vi "p1.vi"() -> ()   [LabVIEW 2023, in "d21.lvlib"]
uses:
  d21.lvlib
  AOC/AOC.lvlib
panel:
  out "Answer":i32
  in  "Example":string="...........\n.....###.#.\n.###.##..#.\n..#.#...#..\n....#.#....\n.##..S####.\n.##..#...#.\n.......##..\n.##.#.####.\n.##..##.##.\n..........."
  in  "Example":bool
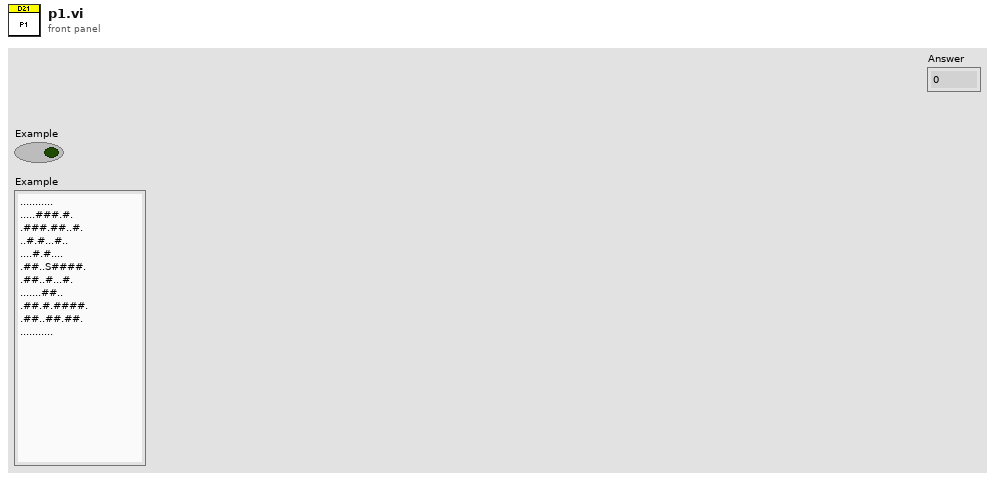
[diagram p1: front panel]
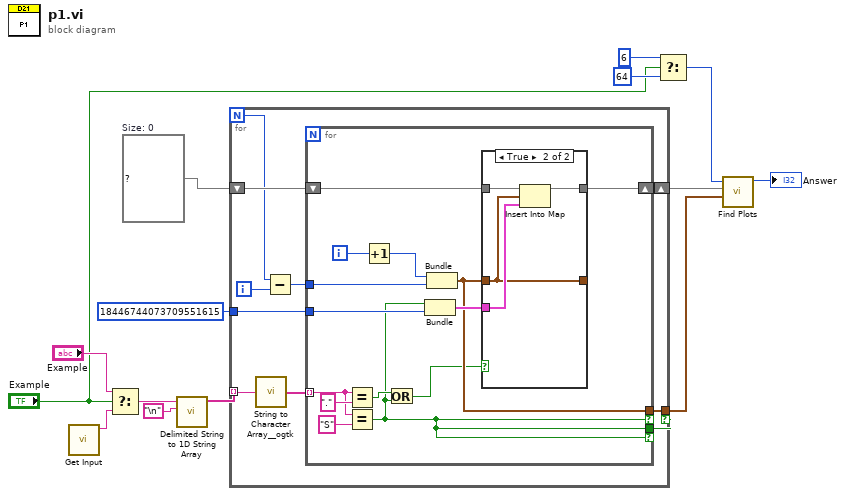
[diagram p0: block diagram]
diagram:
  w8 = map{cluster{i32, i32}, cluster{bool, u64}} {}  # Size: 0
  n1 = call "Get Input.vi"() -> ("Input"=w14:string)  [unwired: 11 in]
  n2 = Select(t="Example", s="Example", f=w14) -> (s? t:f=w13:string)
  n3 = call <vilib>:"Delimited String to 1D String Array.vi"("delimiter"="\n", "delimited string"=w13) -> ("string array"=w10:string[])  [unwired: 9 in]
  n4 = for {
    N -> [w15]
    tunnel: w10 -> [w24] mode=indexing
    tunnel: [w21] -> w3 if=w20
    tunnel: u64 18446744073709551615 -> [w19]
    shift-right: [w17] -> w4
    shift-left: w8 -> [w18]
    i -> [w22]
    n5 = call <userlib>:"String to Character Array__ogtk.vi"("Input String"=w24) -> ("Character Array"=w23:string[])
    n6 = Subtract(x=w15, y=w22) -> (x-y=w16:i32)
    n7 = for {
      tunnel: w23 -> [w37] mode=indexing
      tunnel: w16 -> [w34]
      tunnel: [w28] -> w21 if=w26
      tunnel: [w26] -> w20 if=w26
      tunnel: w19 -> [w33]
      shift-right: [w32] -> w17
      shift-left: w18 -> [w31]
      i -> [w35]
      n8 = Equal?(x=w37, y=".") -> (x = y?=w27:bool)
      n9 = Equal?(x=w37, y="S") -> (x = y?=w26:bool)
      n10 = Increment(x=w35) -> (x+1=w29:i32)
      n11 = Or(x=w27, y=w26) -> (x .or. y?=w25:bool)
      n12 = Bundle(w26, w33) -> (w30:cluster{bool, u64})  [unwired: 1 in]
      n13 = Bundle(w29, w34) -> (w28:cluster{i32, i32})  [unwired: 1 in]
      n14 = case shown="True" w25 {
        tunnel: [w40 w44] -> w32
        tunnel: w31 -> [w40 w43]
        tunnel: w28 -> [w39 w41]
        tunnel: w30 -> [_ w42]
        tunnel: [w39 w41] -> _
        frame False {
        }
        frame True {
          n15 = Insert Into Map(map in=w43, key=w41, value=w42) -> (map out=w44:map{cluster{i32, i32}, cluster{bool, u64}})  [unwired: 2 out]
        }
      }
    }
  }
  n16 = Select(t=6, s="Example", f=64) -> (s? t:f=w5:i32)
  n17 = call "Find Plots.vi"("Start"=w3, "Map"=w4, "Steps"=w5) -> ("Answer"=→"Answer":u64)  [unwired: 8 in]
